vi "Command Parser.vi"(10 "Task IN":string, 11 "Numeric":i32) -> (2 "Task Out":string)   [LabVIEW 2025]
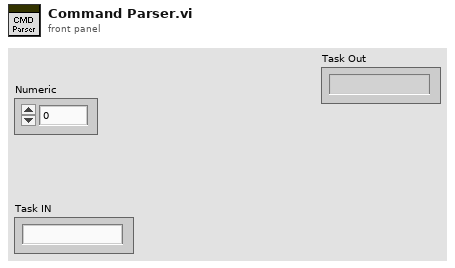
[diagram p1: front panel]
types:
  T1 = enum16{"*IDN?", "CONT MODE?", "CONT MODE PC", "CONT MODE INT", "SOUR VOLT ", "SOUR CURR ", "MEAS VOLT?", "MEAS CURR?", "MEAS AUX1?", "MEAS AUX2?", "MEAS TEMP?"}
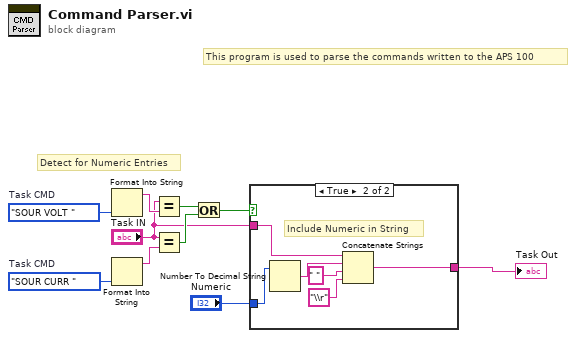
[diagram p0: block diagram]
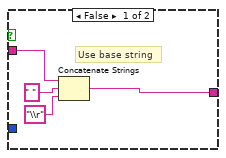
[diagram p2: hidden frame]
diagram:
  w4 = T1."SOUR CURR "  # Task CMD
  w6 = T1."SOUR VOLT "  # Task CMD
  # "This program is used to parse the commands written to the APS 100"
  # "Detect for Numeric Entries"
  n1 = Format Into String(w6) -> (resulting string=w5:string)  [unwired: 3 in, 1 out]
  n2 = Format Into String(w4) -> (resulting string=w3:string)  [unwired: 3 in, 1 out]
  n3 = Equal?(x="Task IN", y=w5) -> (x = y?=w8:bool)
  n4 = Equal?(x="Task IN", y=w3) -> (x = y?=w7:bool)
  n5 = Or(x=w8, y=w7) -> (x .or. y?=w2:bool)
  n6 = case shown="True" w2 {
    tunnel: "Numeric" -> [_ w18]
    tunnel: [w12 w16] -> w9
    tunnel: "Task IN" -> [w11 w15]
    frame False {
      # "Use base string"
      n7 = Concatenate Strings(w11, " " ("string"), "\\r" ("string")) -> (w12:string)
    }
    frame True {
      # "Include Numeric in String"
      n8 = Number To Decimal String(number=w18) -> (decimal integer string=w17:string)  [unwired: 1 in]
      n9 = Concatenate Strings(w15, w17, " " ("string"), "\\r" ("string")) -> (w16:string)
    }
  }
  "Task Out" <- w9
